vi "Math-Column Std Dev.vi"(1 "2D Array":dbl[][](array[numeric])) -> (0 "Column means":dbl[](array[numeric]))   [LabVIEW 2020]
uses:
  <vilib>/Analysis/NI_AALBase.lvlib
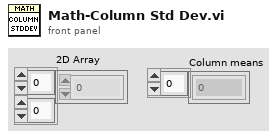
[diagram p1: front panel]
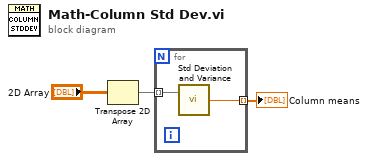
[diagram p0: block diagram]
diagram:
  n1 = Transpose 2D Array(2D array="2D Array") -> (transposed array=w2:dbl[][])
  n2 = for {
    tunnel: w2 -> [w5] mode=indexing
    tunnel: [w4] -> w1 mode=indexing
    n3 = call <vilib>:"Std Deviation and Variance.vi"("X"=w5) -> ("standard deviation"=w4:dbl)  [unwired: 1 in, 2 out]
  }
  "Column means" <- w1
